vi "(SubVI)Scope_Peak to Peak.vi"(7 "Activated Ch":bool[](array[boolean]), 11 "Data In":dbl[][](array[numeric])) -> (3 "PP":T1 {"S3_Value" format="%#_g g"; "S2_Value" format="%#_g g"; "S1_Value" format="%#_g g"})   [LabVIEW 2020]
uses:
  Controls/(Ctrl)Scope_Peak to Peak.ctl
  Controls/(Ctrl)Scope_Sensor Axis.ctl
panel:
  # "Sensor 1"
  # "Sensor 2"
  # "Sensor 3"
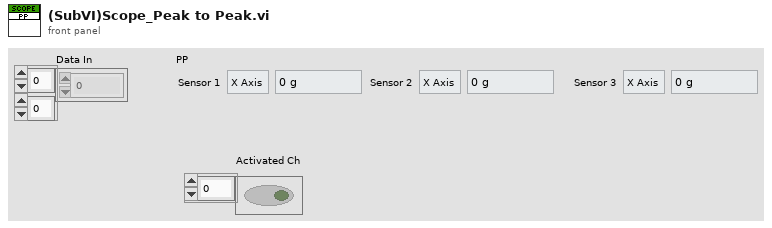
[diagram p1: front panel]
types:
  T1 = typedef "(Ctrl)Scope_Peak to Peak.ctl" = cluster{"S1_Axis":T2, "S1_Value":dbl, "S2_Axis":T2, "S2_Value":dbl, "S3_Axis":T2, "S3_Value":dbl}
  T2 = typedef "(Ctrl)Scope_Sensor Axis.ctl" = enum16{"X Axis", "Y Axis", "Z Axis"}
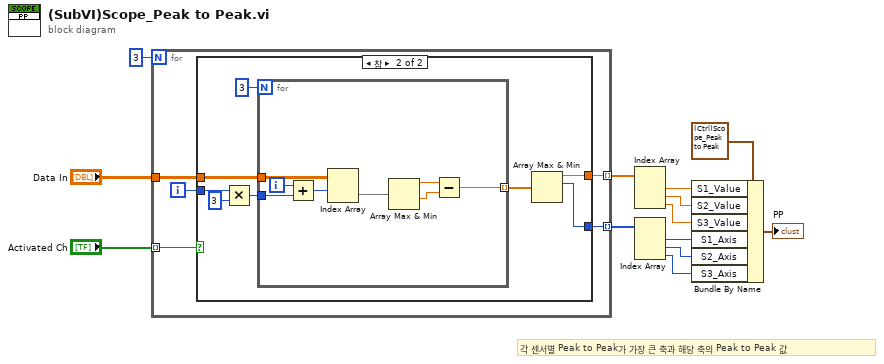
[diagram p0: block diagram]
diagram:
  # "각 센서별 Peak to Peak가 가장 큰 축과 해당 축의 Peak to Peak 값"
  n1 = for {
    N: 3 -> [_]
    tunnel: "Data In" -> [w18]
    tunnel: [w16] -> w11 mode=indexing
    tunnel: [w15] -> w12 mode=indexing
    tunnel: "Activated Ch" -> [w14] mode=indexing
    i -> [w17]
    n2 = case shown="참" w14 {
      tunnel: w18 -> [_ w26]
      tunnel: w17 -> [_ w25]
      tunnel: [_ w21] -> w16
      tunnel: [_ w20] -> w15
      frame False {
      }
      frame True {
        n3 = Multiply(x=w25, y=3) -> (x*y=w23:i32)
        n4 = for {
          N: 3 -> [_]
          tunnel: w26 -> [w34]
          tunnel: w23 -> [w33]
          tunnel: [w27] -> w22 mode=indexing
          i -> [w32]
          n5 = Add(x=w32, y=w33) -> (x+y=w31:i32)
          n6 = Index Array(array=w34, index (row)=w31) -> (element=w30:dbl[])  [unwired: 1 in]
          n7 = Array Max & Min(array=w30) -> (max value=w29:dbl, min value=w28:dbl)  [unwired: 2 out]
          n8 = Subtract(x=w29, y=w28) -> (x-y=w27:dbl)
        }
        n9 = Array Max & Min(array=w22) -> (max value=w20:dbl, max index (indices)=w21:i32)  [unwired: 2 out]
      }
    }
  }
  n10 = Index Array(array=w12) -> (element #1=w9:dbl, element #2=w8:dbl, element #3=w7:dbl)  [unwired: 3 in]
  n11 = Index Array(array=w11) -> (element #1=w6:i32, element #2=w5:i32, element #3=w4:i32)  [unwired: 3 in]
  n12 = Bundle By Name(cluster=T1 {"S1_Axis"=enum."X Axis", "S1_Value"=0.0, "S2_Axis"=enum."X Axis", "S2_Value"=0.0, "S3_Axis"=enum."X Axis", "S3_Value"=0.0} ("Graph_PP"), "S1_Value"=w9, "S2_Value"=w8, "S3_Value"=w7, "S1_Axis"=w6, "S2_Axis"=w5, "S3_Axis"=w4) -> (→"PP":T1)
